vi "Compute_Install_Paths.vi"(8 "error in (no error)":errorcluster, 11 "Installer in":refnum<class "Installer.lvclass">) -> (0 "error out":errorcluster, 3 "Installer out":refnum<class "Installer.lvclass">)   [LabVIEW 2020, in "Installer.lvclass"]
uses:
  <vilib>/AppBuilder/IB_Classes/Installer/Installer.lvclass
  <vilib>/AppBuilder/IB_Classes/Installer/Installer.lvclass/Installer.ctl
  <vilib>/AppBuilder/IB_Classes/Destination/IB_Destination.lvclass
  <vilib>/AppBuilder/IB_Classes/Source/IB_Source.lvclass
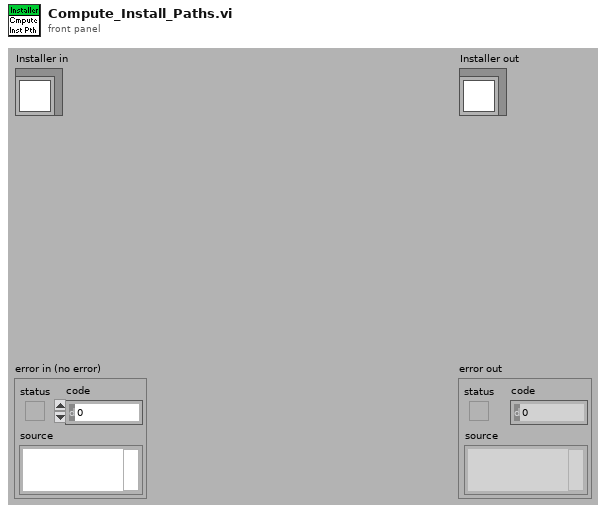
[diagram p1: front panel]
types:
  T1 = typedef "IB_Destination.ctl" = cluster{"name":string, "unlock":bool, "parentTag":string, "destTag":string, "eng_installPath":string}
  T2 = typedef "IB_Source.ctl" = cluster{"name":string, "sourceTag":string, "destTag":string, "path":path, "eng_installPath":string, "UI_inBuild?":bool, "str ref?":bool}
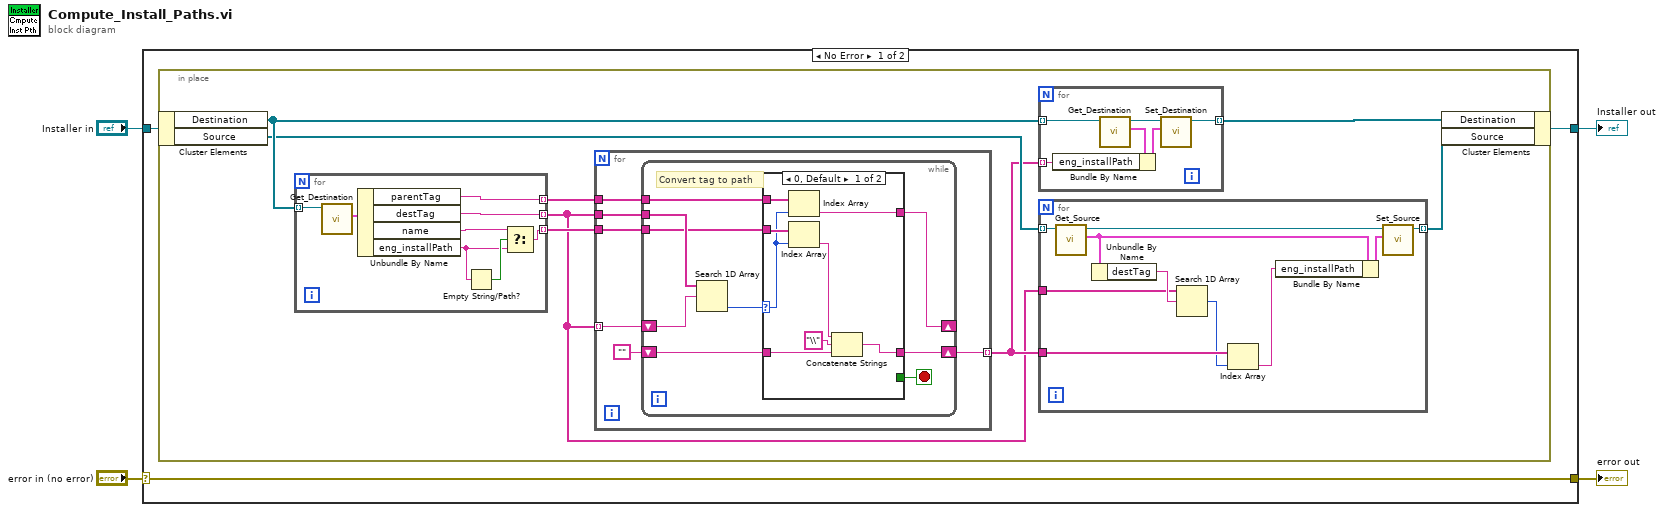
[diagram p0: block diagram]
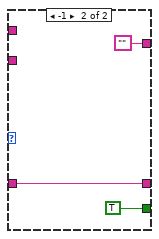
[diagram p2: hidden frame]
diagram:
  n1 = case shown="No Error" "error in (no error)" {
    selector: "error in (no error)" -> [w7 w67]
    tunnel: [w7 w67] -> w3
    tunnel: [w5 w66] -> w1
    tunnel: "Installer in" -> [w6 w66]
    frame No Error {
      n2 = in-place {
        n3 = in-place-cluster #1(w6) -> ("Destination"=w13:refnum<class "IB_Destination.lvclass">[], "Source"=w11:refnum<class "IB_Source.lvclass">[])
        n4 = for {
          tunnel: [w65] -> w15 mode=indexing
          tunnel: [w64] -> w8 mode=indexing
          tunnel: [w58] -> w14 mode=indexing
          tunnel: w13 -> [w62] mode=indexing
          n5 = call <vilib>:"Get_Destination.vi"("IB_Destination in"=w62) -> ("data"=w63:T1)  [unwired: 1 in, 9 out]
          n6 = Unbundle By Name(w63) -> ("parentTag"=w65:string, "destTag"=w64:string, "name"=w59:string, "eng_installPath"=w60:string)
          n7 = Empty String/Path?(string/path=w60) -> (empty?=w61:bool)
          n8 = Select(t=w59, s=w61, f=w60) -> (s? t:f=w58:string)
        }
        n9 = for {
          tunnel: w15 -> [w36]
          tunnel: w8 -> [w35]
          tunnel: w14 -> [w34]
          tunnel: w8 -> [w33] mode=indexing
          tunnel: [w32] -> w9 mode=indexing
          n10 = while {
            tunnel: w36 -> [w44]
            tunnel: w34 -> [w43]
            shift-right: [w39] -> w32
            shift-left: "" -> [w40]
            shift-right: [w42] -> _
            shift-left: w33 -> [w46]
            tunnel: w35 -> [w45]
            stop <- w38 stop-if-true
            # "Convert tag to path"
            n11 = Search 1D Array(1D array=w45, element=w46) -> (index of element=w41:i32)  [unwired: 1 out]
            n12 = case shown="0, Default" w41 {
              selector: w41 -> [w52 _]
              tunnel: w44 -> [w53 _]
              tunnel: w43 -> [w54 _]
              tunnel: [w51 ""] -> w42
              tunnel: w40 -> [w48 w57]
              tunnel: [w47 w57] -> w39
              tunnel: [_ TRUE] -> w38
              frame 0, Default {
                n13 = Index Array(array=w53, index=w52) -> (element=w51:string)
                n14 = Index Array(array=w54, index=w52) -> (element=w50:string)
                n15 = Concatenate Strings(w50, "\\" ("string"), w48) -> (w47:string)
              }
              frame -1 {
              }
            }
          }
        }
        n16 = for {
          tunnel: w13 -> [w30] mode=indexing
          tunnel: [w29] -> w12 mode=indexing
          tunnel: w9 -> [w26] mode=indexing
          n17 = call <vilib>:"Get_Destination.vi"("IB_Destination in"=w30) -> ("data"=w28:T1, "IB_Destination out"=w31:refnum<class "IB_Destination.lvclass">)  [unwired: 1 in, 8 out]
          n18 = Bundle By Name(cluster=w28, "eng_installPath"=w26) -> (w27:T1)
          n19 = call <vilib>:"Set_Destination.vi"("data"=w27, "IB_Destination in"=w31) -> ("IB_Destination out"=w29:refnum<class "IB_Destination.lvclass">)  [unwired: 1 in, 8 out]
        }
        n20 = for {
          tunnel: w11 -> [w25] mode=indexing
          tunnel: [w23] -> w10 mode=indexing
          tunnel: w9 -> [w20]
          tunnel: w8 -> [w17]
          n21 = call <vilib>:"Get_Source.vi"("IB_Source in"=w25) -> ("data"=w22:T2, "IB_Source out"=w24:refnum<class "IB_Source.lvclass">)  [unwired: 1 in, 8 out]
          n22 = Unbundle By Name(w22) -> ("destTag"=w18:string)
          n23 = Search 1D Array(1D array=w17, element=w18) -> (index of element=w16:i32)  [unwired: 1 out]
          n24 = Index Array(array=w20, index=w16) -> (element=w19:string)
          n25 = Bundle By Name(cluster=w22, "eng_installPath"=w19) -> (w21:T2)
          n26 = call <vilib>:"Set_Source.vi"("data"=w21, "IB_Source in"=w24) -> ("IB_Source out"=w23:refnum<class "IB_Source.lvclass">)  [unwired: 1 in, 8 out]
        }
        n27 = in-place-cluster #1("Destination"=w12, "Source"=w10) -> (w5:refnum<class "Installer.lvclass">)
      }
    }
    frame Error {
    }
  }
  "error out" <- w3
  "Installer out" <- w1
